vi "H5Pset_cache.vi"(6 "rdcc_w0":dbl, 7 "mdc_nelmts":i32, 8 "error in (no error)":errorcluster, 9 "rdcc_nbytes":u64, 10 "rdcc_nelmts":u64, 11 "HDF5 Property List Ref":T1) -> (0 "error out":errorcluster, 3 "HDF5 Property List Ref out":T1)   [LabVIEW 2017]
doc: "Sets the raw data chunk cache parameters.</dd>\n \n <br />"
uses:
  <vilib>/UPVI/lvhdf5/library.llb/HDF5 Ref.ctl
  <vilib>/UPVI/lvhdf5/hdf5.dll
panel:
  # "LVHDF5 Toolkit\nCopyright (c) 2005-2013 by Jason D. Sommerville\nCopyright (c) 2014 by UPVI, LLC.\n\nThis use and distribution of this file is governed by the terms found in \nLICENSE.txt distributed with this toolkit and installed at\n <user.lib>\\_lvhdf5\\LICENSE.txt"
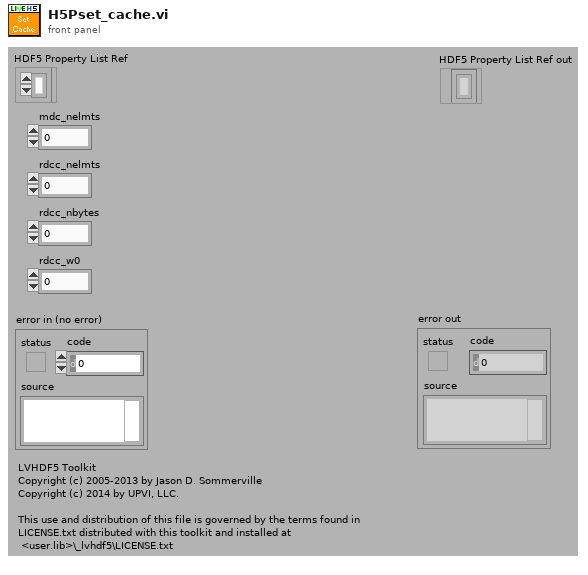
[diagram p1: front panel]
types:
  T1 = typedef "HDF5 Ref.ctl" = refnum<k1>
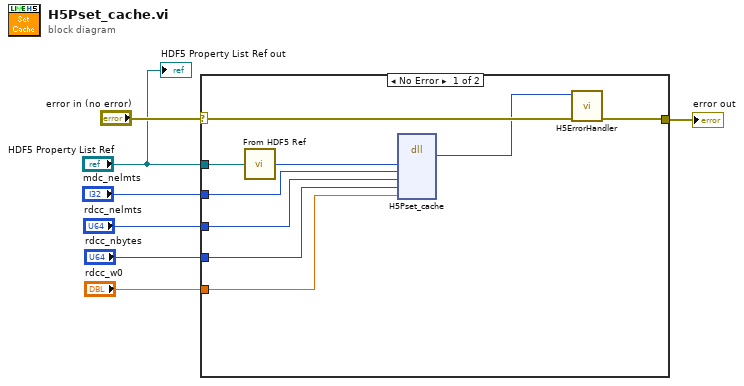
[diagram p0: block diagram]
diagram:
  n1 = case shown="No Error" "error in (no error)" {
    selector: "error in (no error)" -> [w16 w17]
    tunnel: [w15 w17] -> w6
    tunnel: "HDF5 Property List Ref" -> [w14 _]
    tunnel: "mdc_nelmts" -> [w11 _]
    tunnel: "rdcc_nelmts" -> [w10 _]
    tunnel: "rdcc_nbytes" -> [w9 _]
    tunnel: "rdcc_w0" -> [w8 _]
    frame No Error {
      n2 = call <vilib>:"From HDF5 Ref.vi"("HDF5 Ref"=w14) -> ("I32"=w13:i32)
      n3 = dll-call lib="C:/Program Files/National Instruments/LabVIEW 2017/vi.lib/UPVI/lvhdf5/hdf5.dll" fn="H5Pset_cache"("plist_id"=w13, "mdc_nelmts"=w11, "rdcc_nelmts"=w10, "rdcc_nbytes"=w9, "rdcc_w0"=w8) -> ("return type"=w12:i32)  [unwired: 8 in, 2 out]
      n4 = call <vilib>:"H5ErrorHandler.vi"("error in (no error)"=w16, "herr_t"=w12) -> ("error out"=w15:errorcluster)  [unwired: 3 in, 4 out]
    }
    frame Error {
    }
  }
  "error out" <- w6
  "HDF5 Property List Ref out" <- "HDF5 Property List Ref"
